vi "imt.vi"() -> ()   [LabVIEW 2015]
uses:
  Framework/test_system/pdbm_test_system.lvlib
panel:
  in  "measure":bool
  in  "updateFirmw":bool
  in  "cfgDevice":bool
  in  "cfgHrdw":bool
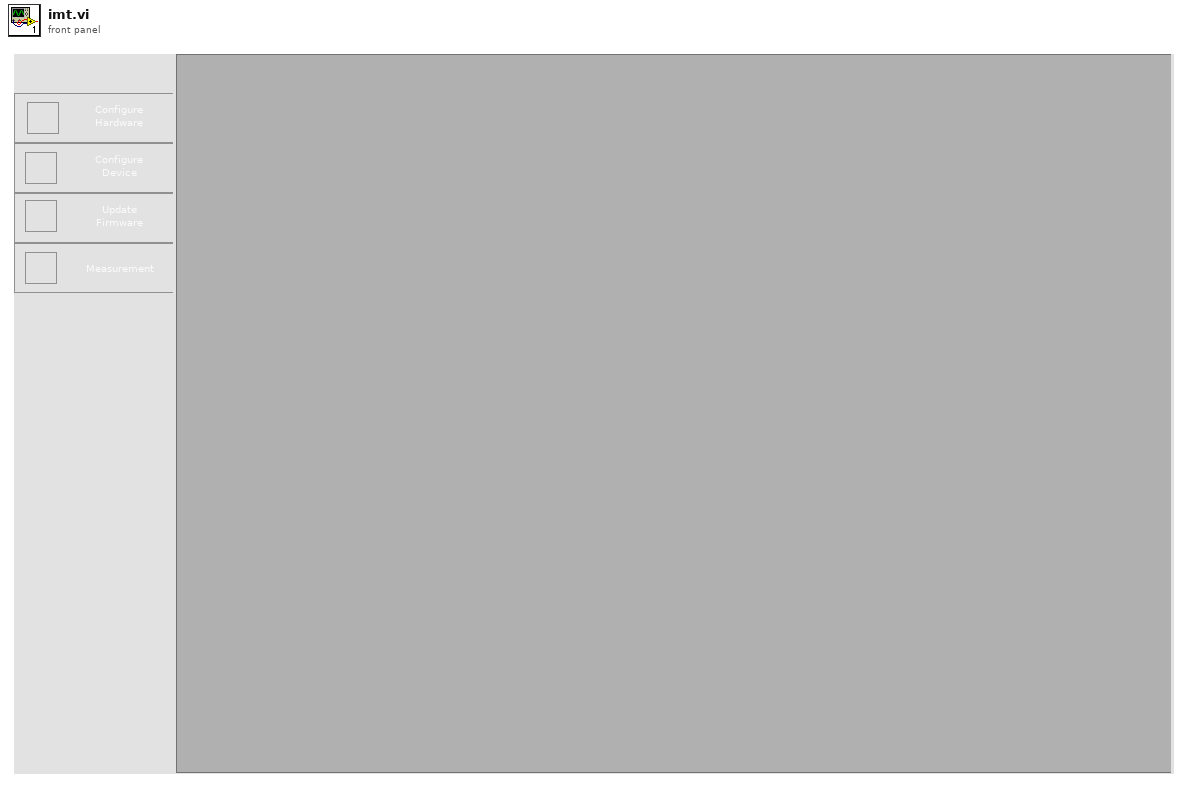
[diagram p1: front panel]
types:
  T1 = enum32{"invalid app kind", "Development System", "Run Time System", "Student Edition", "Embedded LabVIEW", "Evaluation", "Custom"}
  T2 = cluster{"pdbm_testsys_reg_fd_event":refnum<event-registration>, "imt_loadtask_event":refnum<event-registration>}
  T3 = cluster{"imt_testsys_reqst_event":refnum<user-event>, "imt_testsys_fd_event":refnum<user-event>, "imt_loadtask_reg_event":refnum<user-event>}
  T4 = cluster{"imt_testsys_reqst_event":refnum<user-event>, "imt_testsys_fd_event":refnum<user-event>}
  T5 = typedef "imt_app_cmd.ctl" = enum16{"unknown", "configHardware", "configDevice", "updateFirmware", "measurement"}
  T6 = typedef "pdbm_test_system.lvlib/pdbm_testsystem_feedback_data.ctl" = cluster{"TaskName":string, "Request":string, "Data":variant}
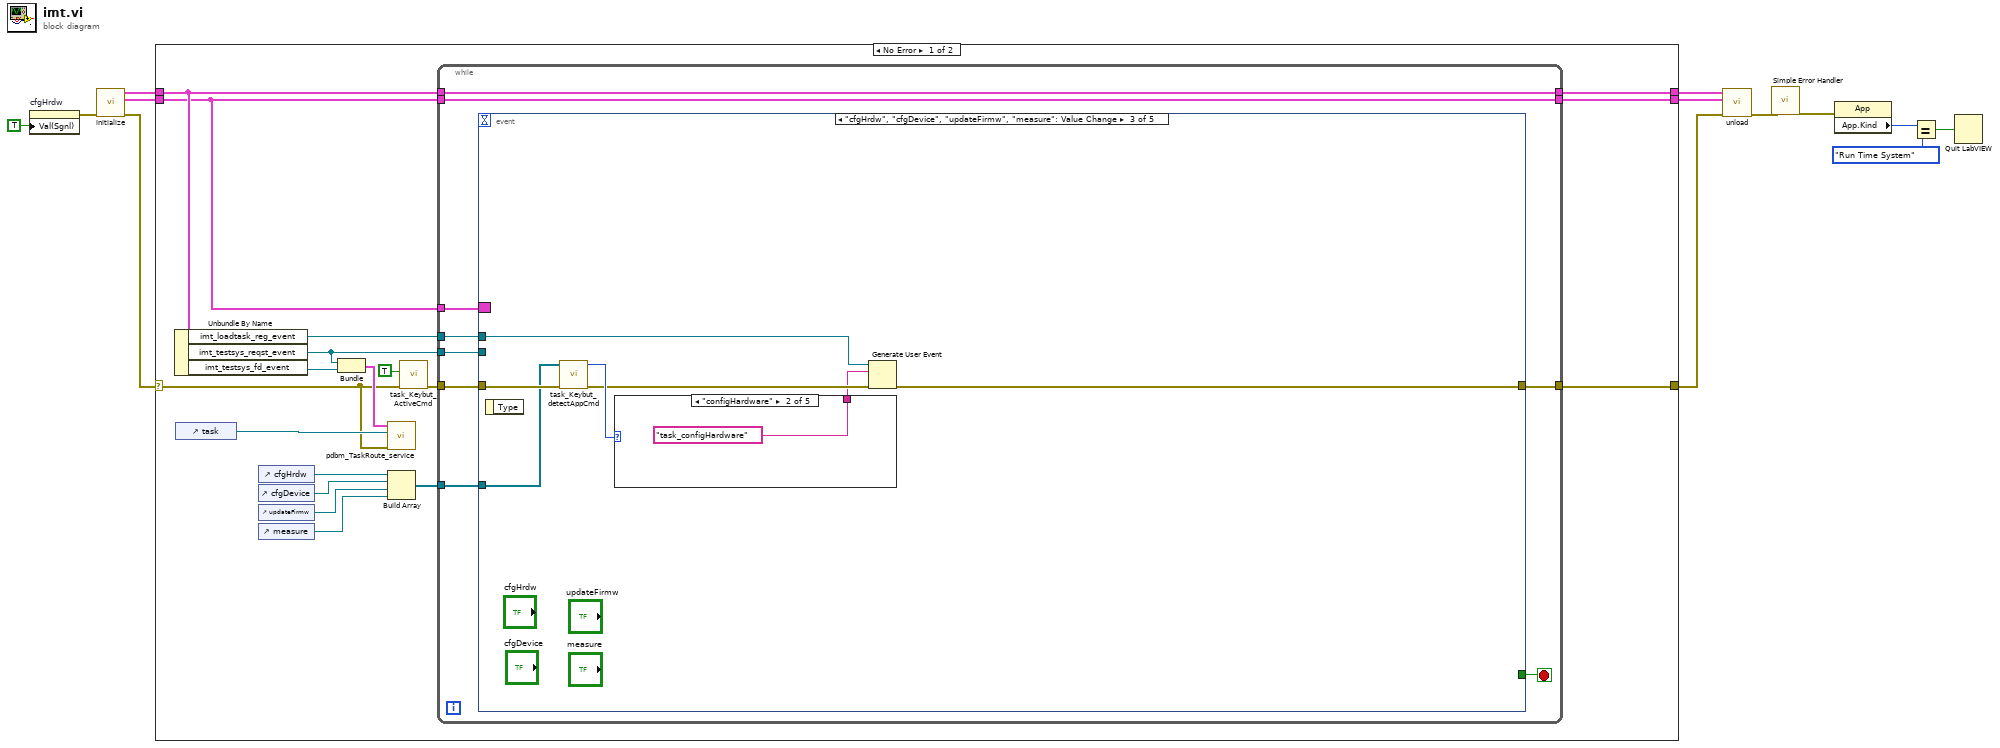
[diagram p0: block diagram]
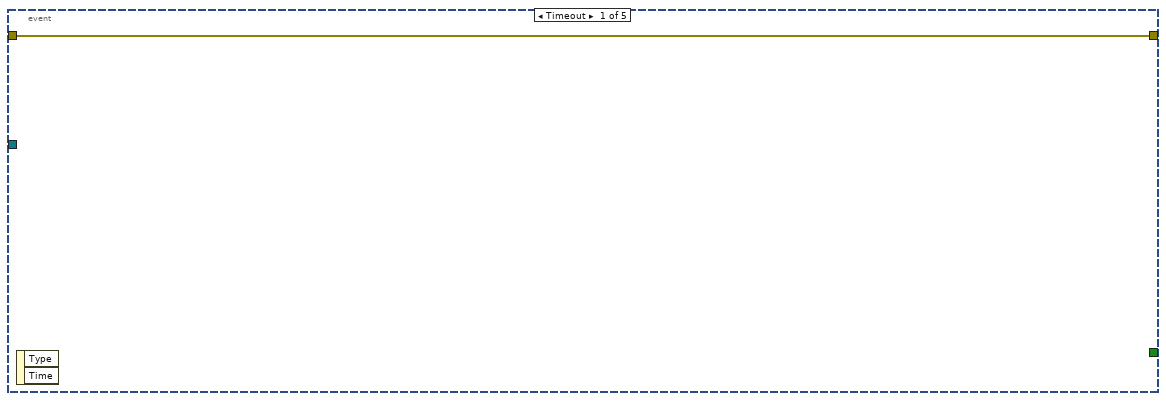
[diagram p2: hidden frame]
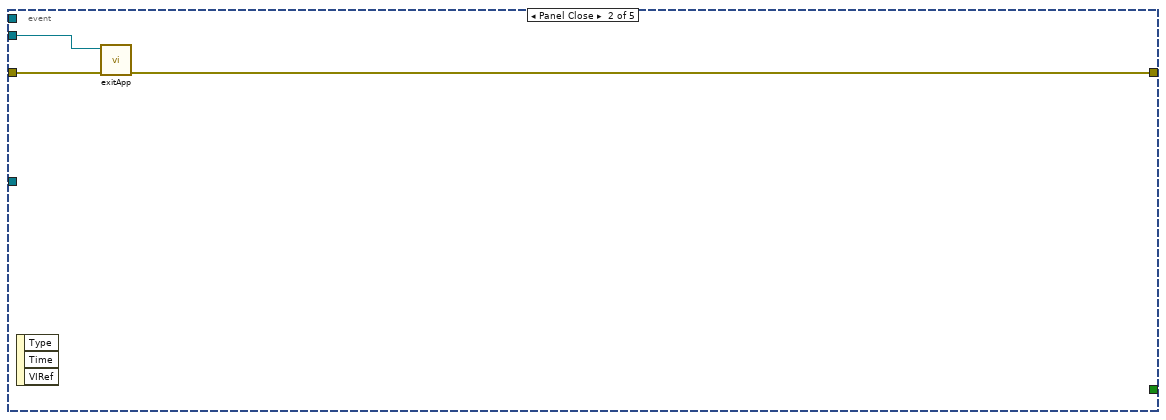
[diagram p3: hidden frame]
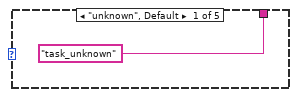
[diagram p4: hidden frame]
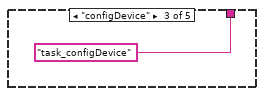
[diagram p5: hidden frame]
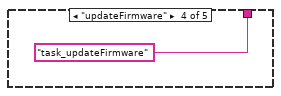
[diagram p6: hidden frame]
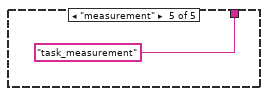
[diagram p7: hidden frame]
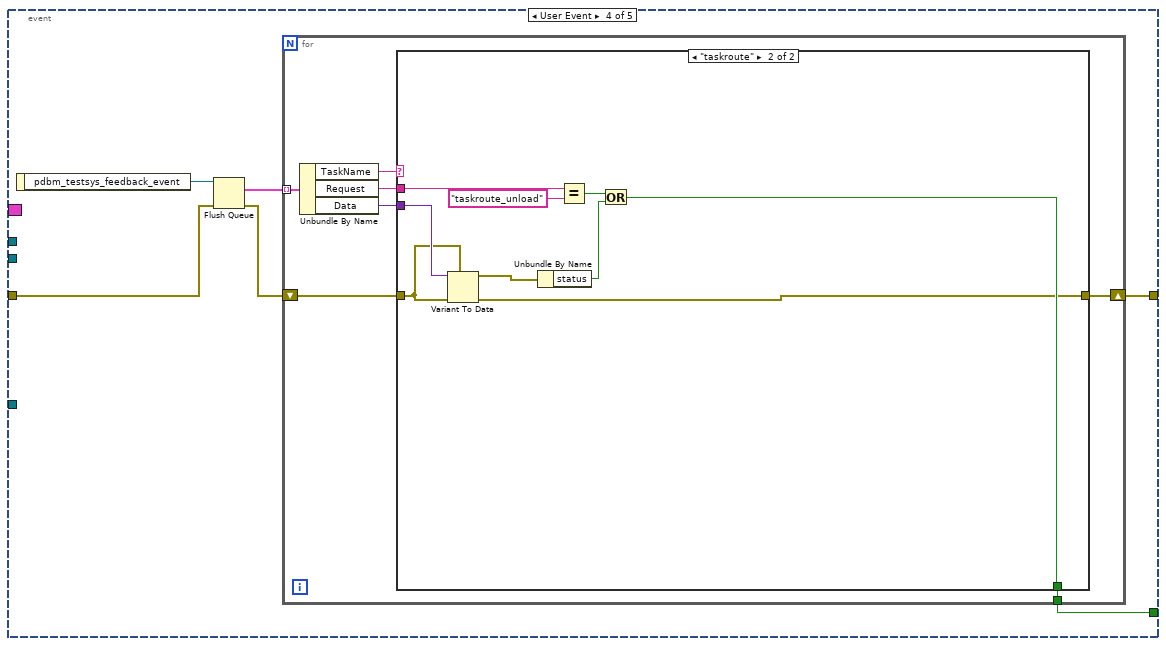
[diagram p8: hidden frame]
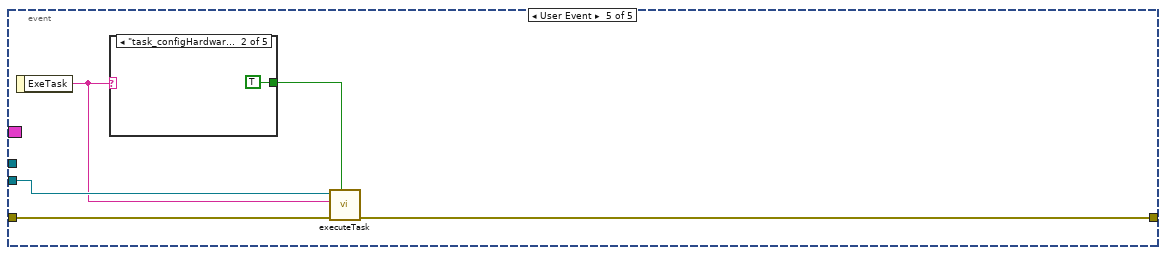
[diagram p10: hidden frame]
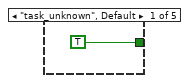
[diagram p11: hidden frame]
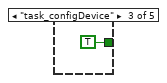
[diagram p12: hidden frame]
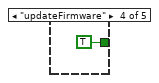
[diagram p13: hidden frame]
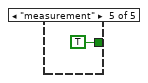
[diagram p14: hidden frame]
diagram:
  n1 = property on="cfgHrdw" class="Bool (strict)"("Val(Sgnl)"=TRUE ("Value (Signaling)")) -> (error out=w2:errorcluster)  [unwired: 2 in, 1 out]
  n2 = call "initialize.vi"("error in (no error)"=w2) -> ("error IO"=w11:errorcluster, "pdbm_testsys_reg_event"=w13:T2, "pdbm_testsys_event"=w12:T3)  [unwired: 8 in]
  n3 = case shown="No Error" w11 {
    selector: w11 -> [w15 w90]
    tunnel: w13 -> [w24 w91]
    tunnel: w12 -> [w27 w92]
    tunnel: [w30 w92] -> w10
    tunnel: [w29 w91] -> w9
    tunnel: [w28 w90] -> w8
    frame No Error {
      n4 = Unbundle By Name(w27) -> ("imt_loadtask_reg_event"=w23:refnum<user-event>, "imt_testsys_reqst_event"=w17:refnum<user-event>, "imt_testsys_fd_event"=w26:refnum<user-event>)
      n5 = control-ref of="task"() -> (w31:refnum<vi>)
      n6 = control-ref of="cfgHrdw"() -> (w22:refnum<vi>)
      n7 = control-ref of="cfgDevice"() -> (w21:refnum<vi>)
      n8 = control-ref of="updateFirmw"() -> (w20:refnum<vi>)
      n9 = control-ref of="measure"() -> (w19:refnum<vi>)
      n10 = Bundle("imt_testsys_reqst_event"=w17, "imt_testsys_fd_event"=w26) -> (w25:T4)  [unwired: 1 in]
      n11 = call "pdbm_TaskRoute_service.vi"("error in (no error)"=w15, "TaskDisplay"=w31, "pdbm_testsys_event"=w25) -> ()  [unwired: 9 in]
      n12 = Build Array(w22, w21, w20, w19) -> (w18:refnum<vi>[])
      n13 = call "task_Keybut_ActiveCmd.vi"("error in (no error)"=w15, "update"=TRUE) -> ("error out"=w16:errorcluster)  [unwired: 8 in, 1 out]
      n14 = while {
        tunnel: w27 -> [w35]
        tunnel: w16 -> [w39]
        tunnel: w24 -> [w38]
        tunnel: [w35] -> w30
        tunnel: [w38] -> w29
        tunnel: w24 -> [w37]
        tunnel: [w36] -> w28
        tunnel: w23 -> [w34]
        tunnel: w18 -> [w33]
        tunnel: w17 -> [w32]
        stop <- w40 stop-if-true
        n15 = event shown="[2] \"cfgHrdw\", \"cfgDevice\", \"updateFirmw\", \"measure\": Value Change" {
          selector: w37 -> [_ _ _ _ _]
          dyn-events: _ -> [_ _ _ _ _]
          timeout: _ -> [_ _ _ _ _]
          tunnel: [_ _ _ w57 _] -> w40
          tunnel: w39 -> [w41 w44 w51 w61 w84]
          tunnel: [w41 w43 w45 w58 w82] -> w36
          tunnel: w34 -> [_ _ w48 _ _]
          tunnel: w33 -> [_ _ w50 _ _]
          tunnel: w32 -> [_ w42 _ _ w83]
          event Timeout {
            n16 = event-data() -> ()  [unwired: 1 in, 2 out]
          }
          event Panel Close {
            n17 = event-data() -> ()  [unwired: 1 in, 3 out]
            n18 = call "exitApp.vi"("error in (no error)"=w44, "pdbm_testsys_reqst_event"=w42) -> ("error IO"=w43:errorcluster)  [unwired: 8 in, 1 out]
          }
          event "cfgHrdw", "cfgDevice", "updateFirmw", "measure": Value Change {
            n19 = event-data() -> ()  [unwired: 1 in, 1 out]
            n20 = call "task_Keybut_detectAppCmd.vi"("error in (no error)"=w51, "Cmd Ref in"=w50) -> ("error IO"=w47:errorcluster, "AppCmd"=w49:T5)  [unwired: 8 in]
            n21 = case shown="\"configHardware\"" w49 {
              tunnel: ["task_unknown" "task_configHardware" "task_configDevice" "task_updateFirmware" "task_measurement"] -> w46
              frame "unknown", Default {
              }
              frame "configHardware" {
              }
              frame "configDevice" {
              }
              frame "updateFirmware" {
              }
              frame "measurement" {
              }
            }
            n22 = Generate User Event(user event=w48, event data cluster=w46, error in=w47) -> (error out=w45:errorcluster)  [unwired: 1 in, 1 out]
          }
          event User Event {
            n23 = event-data() -> ("pdbm_testsys_feedback_event"=w62:refnum<queue>)  [unwired: 1 in]
            n24 = Flush Queue(queue=w62, error in (no error)=w61) -> (remaining elements=w60:T6[], error out=w59:errorcluster)  [unwired: 1 out]
            n25 = for {
              tunnel: w60 -> [w69] mode=indexing
              shift-right: [w64] -> w58
              shift-left: w59 -> [w65]
              tunnel: [w63] -> w57
              n26 = Unbundle By Name(w69) -> ("TaskName"=w68:string, "Request"=w67:string, "Data"=w66:variant)
              n27 = case shown="\"taskroute\"" w68 {
                tunnel: w67 -> [_ w76]
                tunnel: w66 -> [_ w79]
                tunnel: w65 -> [w70 w78]
                tunnel: [w70 w71] -> w64
                tunnel: [_ w72] -> w63
                frame "False", Default {
                }
                frame "taskroute" {
                  n28 = Variant To Data(error in=w78, type=w78, Variant=w79) -> (data=w77:errorcluster, error out=w71:errorcluster)
                  n29 = Unbundle By Name(w77) -> ("status"=w73:bool)
                  n30 = Equal?(x=w76, y="taskroute_unload") -> (x = y?=w74:bool)
                  n31 = Or(x=w74, y=w73) -> (x .or. y?=w72:bool)
                }
              }
            }
          }
          event User Event {
            n32 = event-data() -> ("ExeTask"=w81:string)  [unwired: 1 in]
            n33 = case shown="\"task_configHardware\"" w81 {
              tunnel: [TRUE TRUE TRUE TRUE TRUE] -> w80
              frame "task_unknown", Default {
              }
              frame "task_configHardware" {
              }
              frame "task_configDevice" {
              }
              frame "updateFirmware" {
              }
              frame "measurement" {
              }
            }
            n34 = call "executeTask.vi"("VisibleTask?"=w80, "error in (no error)"=w84, "Task"=w81, "pdbm_testsys_reqst_event"=w83) -> ("error IO"=w82:errorcluster)  [unwired: 6 in, 1 out]
          }
        }
      }
    }
    frame Error {
    }
  }
  n35 = call "unload.vi"("error in (no error)"=w8, "imt_testsys_reg_event"=w9, "imt_testsys_event"=w10) -> ("error out"=w7:errorcluster)  [unwired: 8 in]
  n36 = call <vilib>:"Simple Error Handler.vi"("error in (no error)"=w7) -> ("error out"=w6:errorcluster)  [unwired: 4 in, 4 out]
  n37 = property class="App"(error in=w6) -> ("App.Kind"=w5:T1)  [unwired: 1 in, 2 out]
  n38 = Equal?(x=w5, y=T1."Run Time System") -> (x = y?=w3:bool)
  n39 = Quit LabVIEW(quit? (T)=w3) -> ()
